vi "Timer.vi"(0 "t0 (ms)":u32, 1 "error in (no error)":errorcluster) -> (12 "elapsed [or start time] (ms)":u32, 14 "t now (ms)":u32, 15 "error out":errorcluster)   [LabVIEW 2017]
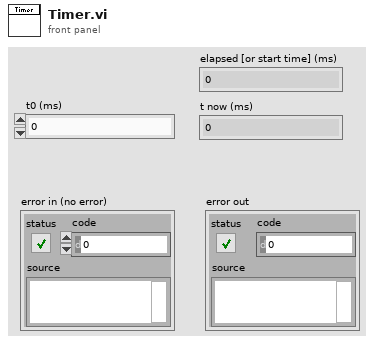
[diagram p1: front panel]
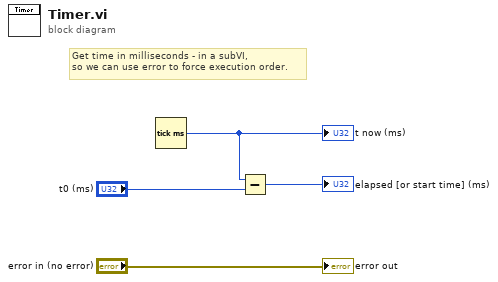
[diagram p0: block diagram]
diagram:
  # "Get time in milliseconds - in a subVI,\nso we can use error to force execution order."
  n1 = Tick Count (ms)() -> (millisecond timer value=w1:u32)
  "t now (ms)" <- w1
  n2 = Subtract(x=w1, y="t0 (ms)") -> (x-y=→"elapsed [or start time] (ms)":u32)
  "error out" <- "error in (no error)"
